vi "Fluke 5080 AC DC Voltage Calibrator.vi"() -> ()   [LabVIEW 2012]
doc: "This example shows how to configure the calibrator to ac/dc voltage output mode."
uses:
  <instrlib>/Fluke 5080/Fluke 5080.lvlib
panel:
  in  "Output Impedance (50 Ohm)":i32=50
  in  "Serial Configuration":T1={"Baud Rate"=9600, "Parity"=0, "Data Bits"=8, "Stop Bits"=10, "Flow Control"=0} {"Flow Control" items=["None", "XON/XOFF", "RTS/CTS", "XON/XOFF & RTS/CTS", "DTR/DSR", "XON/XOFF & DTR/DSR"]; "Stop Bits" items=["1.0"=10, "1.5"=15, "2.0"=20]; "Data Bits" items=["7"=7, "8"=8]; "Parity" items=["None", "Odd", "Even", "Mark", "Space"]; "Baud Rate" items=["300"=300, "600"=600, "1200"=1200, "2400"=2400, "4800"=4800, "9600"=9600, "19200"=19200]}
  in  "VISA resource name":refnum<visa-resource-name>
  in  "Frequency (50.0 Hertz)":dbl=50.0
  in  "Phase (0.0 Degrees)":dbl
  in  "Primary Voltage (5.0)":dbl=5.0
  in  "Output Type (0: DC Volts)":i32(ring)=1 items=["DC Volts", "AC Volts", "DC Current", "AC Current", "DC Power", "AC Power", "Dual DC Volts", "Dual AC Volts", "Resistance"]
  in  "Earth Ground Enabled (T: Enabled)":bool=TRUE
  # "(c) 2010 National Instruments.  ALL RIGHTS RESERVED."
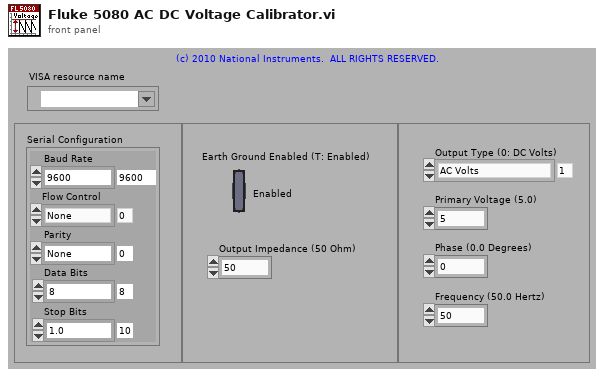
[diagram p1: front panel]
types:
  T1 = cluster{"Baud Rate":u32, "Parity":u16, "Data Bits":u16, "Stop Bits":u16, "Flow Control":u16}
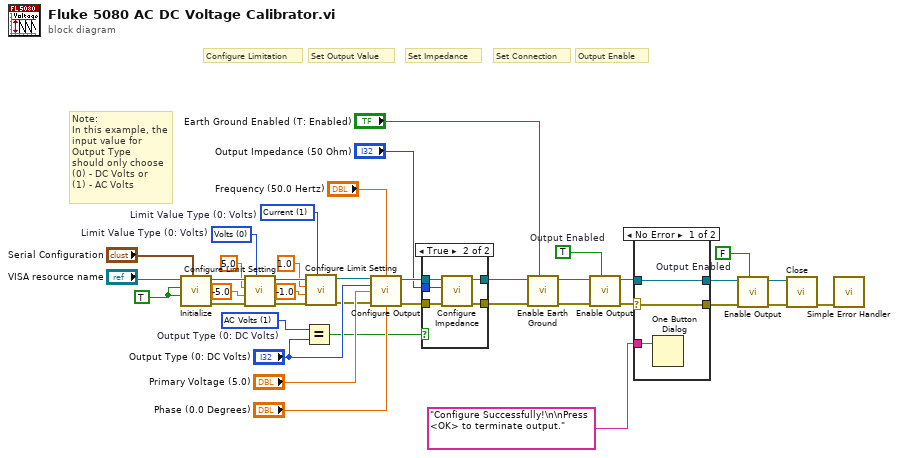
[diagram p0: block diagram]
diagram:
  w5 = 0 items=["Volts", "Current"]  # Limit Value Type (0: Volts)
  w6 = 1 items=["Volts", "Current"]  # Limit Value Type (0: Volts)
  w11 = TRUE  # Output Enabled
  w19 = FALSE  # Output Enabled
  w22 = 1 items=["DC Volts", "AC Volts", "DC Current", "AC Current", "DC Power", "AC Power", "Dual DC Volts", "Dual AC Volts", "Resistance"]  # Output Type (0: DC Volts)
  w39 = TRUE ("Reset (True)")
  # "Set Connection"
  # "Note:\nIn this example, the \ninput value for \nOutput Type\nshould only choose \n(0) - DC Volts or \n(1) - AC Volts"
  # "Output Enable"
  # "Set Impedance"
  # "Set Output Value"
  # "Configure Limitation"
  n1 = call <instrlib>:"Initialize.vi"("Serial Configuration"="Serial Configuration", "Reset (True)"=w39, "ID Query (True)"=w39, "VISA resource name"="VISA resource name") -> ("error out"=w37:errorcluster, "VISA resource name out"=w36:refnum<visa-resource-name>)  [unwired: 1 in, 5 out]
  n2 = call <instrlib>:"Configure Limit Setting.vi"("Limit Value Type (0: Volts)"=w5, "error in (no error)"=w37, "- Limit Value (-5)"=-5.0, "+ Limit Value (5)"=5.0, "VISA resource name"=w36) -> ("error out"=w9:errorcluster, "VISA resource name out"=w10:refnum<visa-resource-name>)  [unwired: 5 out]
  n3 = Equal?(x=w22, y="Output Type (0: DC Volts)") -> (x = y?=w20:bool)
  n4 = call <instrlib>:"Configure Limit Setting.vi"("Limit Value Type (0: Volts)"=w6, "error in (no error)"=w9, "- Limit Value (-5)"=-1.0, "+ Limit Value (5)"=1.0, "VISA resource name"=w10) -> ("error out"=w7:errorcluster, "VISA resource name out"=w8:refnum<visa-resource-name>)  [unwired: 5 out]
  n5 = call <instrlib>:"Configure Output.vi"("VISA resource name"=w8, "Frequency (50.0 Hertz)"="Frequency (50.0 Hertz)", "Output Type (0: DC Volts)"="Output Type (0: DC Volts)", "Primary Voltage (5.0)"="Primary Voltage (5.0)", "error in (no error)"=w7, "Phase (0.0 Degrees)"="Phase (0.0 Degrees)") -> ("VISA resource name out"=w26:refnum<visa-resource-name>, "error out"=w27:errorcluster)  [unwired: 4 in, 4 out]
  n6 = case shown="True" w20 {
    tunnel: [w41 w46] -> w29
    tunnel: [w40 w45] -> w28
    tunnel: w27 -> [w40 w44]
    tunnel: w26 -> [w41 w43]
    tunnel: "Output Impedance (50 Ohm)" -> [_ w42]
    frame False {
    }
    frame True {
      n7 = call <instrlib>:"Configure Impedance.vi"("error in (no error)"=w44, "Output Impedance (50 Ohm)"=w42, "VISA resource name"=w43) -> ("error out"=w45:errorcluster, "VISA resource name out"=w46:refnum<visa-resource-name>)  [unwired: 7 out]
    }
  }
  n8 = call <instrlib>:"Enable Earth Ground.vi"("Earth Ground Enabled (T: Enabled)"="Earth Ground Enabled (T: Enabled)", "error in (no error)"=w28, "VISA resource name"=w29) -> ("error out"=w23:errorcluster, "VISA resource name out"=w24:refnum<visa-resource-name>)  [unwired: 7 out]
  n9 = call <instrlib>:"Enable Output.vi"("Output Enabled (T: Enable)"=w11, "error in (no error)"=w23, "VISA resource name"=w24) -> ("error out"=w14:errorcluster, "VISA resource name out"=w15:refnum<visa-resource-name>)  [unwired: 7 out]
  n10 = case shown="No Error" w14 {
    selector: w14 -> [w48 w50]
    tunnel: "Configure Successfully!\n\nPress <OK> to terminate output." ("message") -> [w49 _]
    tunnel: [w48 w50] -> w16
    tunnel: [w47 w51] -> w17
    tunnel: w15 -> [w47 w51]
    frame No Error {
      n11 = One Button Dialog(message=w49) -> ()  [unwired: 2 out]
    }
    frame Error {
    }
  }
  n12 = call <instrlib>:"Enable Output.vi"("Output Enabled (T: Enable)"=w19, "error in (no error)"=w16, "VISA resource name"=w17) -> ("error out"=w12:errorcluster, "VISA resource name out"=w13:refnum<visa-resource-name>)  [unwired: 7 out]
  n13 = call <instrlib>:"Close.vi"("error in (no error)"=w12, "VISA resource name"=w13) -> ("error out"=w32:errorcluster)  [unwired: 9 out]
  n14 = call <vilib>:"Simple Error Handler.vi"("error in (no error)"=w32) -> ()  [unwired: 1 in, 8 out]
